vi "RunCount.vi"(1 "TestResultMock In":refnum<class "TestResultMock.lvclass">) -> (0 "Run Count":i32)   [LabVIEW 2019, in "TestSuiteTest.lvlib" / "Support.lvlib" / "TestResultMock.lvclass"]
uses:
  TestResultMock.lvclass
  TestResultMock.lvclass/TestResultMock.ctl
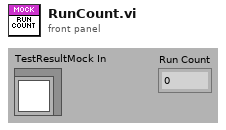
[diagram p1: front panel]
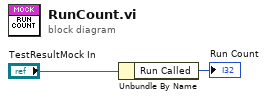
[diagram p0: block diagram]
diagram:
  n1 = Unbundle By Name("TestResultMock In") -> ("Run Called"=→"Run Count":i32)
